vi "Clear Restarted Flag.vi"(8 "error in (no error)":errorcluster, 11 "PLBB in":refnum<class "PL BlackBox Modbus Client.lvclass">) -> (0 "error out":errorcluster, 3 "PLBB out":refnum<class "PL BlackBox Modbus Client.lvclass">)   [LabVIEW 2015, in "PL BlackBox Modbus Client.lvclass"]
doc: "Clears the restarted flag."
uses:
  PL BlackBox Modbus Client.lvclass
  <vilib>/plasmapper/PL Modbus Client/PL Modbus Client.lvclass
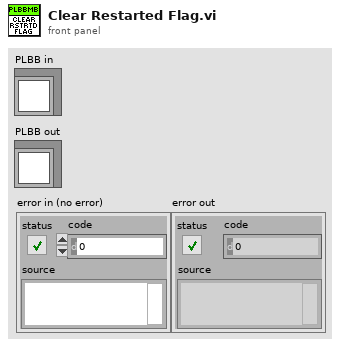
[diagram p1: front panel]
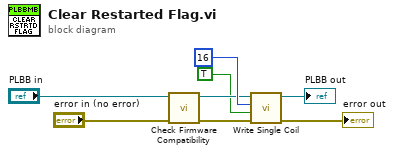
[diagram p0: block diagram]
diagram:
  n1 = call-dynamic "Check Firmware Compatibility.vi"("error in (no error)"="error in (no error)", "PLBB in"="PLBB in") -> ("error out"=w4:errorcluster, "PLBB out"=w5:refnum<class "PL BlackBox Modbus Client.lvclass">)  [unwired: 8 in]
  n2 = call <vilib>:"Write Single Coil.vi"("error in (no error)"=w4, "value"=TRUE, "address"=u16 16, "MODBUS in"=w5) -> ("error out"=→"error out":errorcluster, "MODBUS out"=→"PLBB out":refnum<class "PL BlackBox Modbus Client.lvclass">)  [unwired: 6 in]
